vi "fuse_CAN_tester.vi"() -> ()   [LabVIEW 2010]
uses:
  <vilib>/Platform/TimedLoop/XDataNode/XDataNode.xnode
  <vilib>/Platform/TimedLoop/XDataNode/timing_clust.ctl
  <vilib>/Platform/TimedLoop/XDataNode/nitl_modes.ctl
  <vilib>/Platform/TimedLoop/XDataNode/wakeup.ctl
  <vilib>/Platform/TimedLoop/XDataNode/XDNodeRunTimeDep.lvlib
panel:
  in  "Save Params":bool
  in  "Frequancy":i32
  out "WD reset":bool
  in  "Clear buffer":bool
  out "Error number":string
  in  "Get Faults":bool
  out "FF OC":bool
  out "Comperator OC":bool
  out "ADC OC":bool
  in  "Params Menu":u8(ring) items=["Address", "Interval Period", "Nm Of Retries", "On time", "Save Parameters"]
  in  "Send Param":bool
  in  "Repeat Command":bool
  in  "Send":bool
  in  "Command Menu":u8(ring) items=["Status"=0, "ADC Reading"=1, "Isc threshold"=2, "Vin Vout"=15, "RESET FF"=3, "Up Time"=5, "Interval Period"=6, "Nm Of Retries"=7, "On time"=8, "Version"=10, "Temperature"=16]
  out "RT (Ohms)":dbl
  out "Temp (C)":dbl
  out "Vout [V]":dbl
  out "Vin [V]":dbl
  in  "Address":u32
  in  "Interval Period":u32
  in  "Nm. Retries":u32
  in  "On Time [us]":u32
  out "On Time [us]":u32
  out "Nm. Retries":u32
  out "Interval [ms]":u32
  out "Up Time":u32
  out "Fuse Current [A]":dbl
  out "ADC Reading":u32
  out "Isc [A]":dbl
  out "Timeout":bool
  out "R Sense [m]":dbl
  out "Fuse Status":bool
  in  "Clear":bool
  out "Command Buffer":string
  out "status":bool
  out "Message List":string
  in  "Open":bool
  in  "Close":bool
  in  "Quit":bool
  in  "Send Message":bool
  in  "Bit Rate":string="250"
  out "Handle":i32
  in  "Data":u8 format="%x"
  in  "Data 2":u8 format="%x"
  in  "Data 3":u8 format="%x"
  in  "Data 4":u8 format="%x"
  in  "Data 5":u8 format="%x"
  in  "Data 6":u8 format="%x"
  in  "Data 7":u8 format="%x"
  in  "Data 8":u8 format="%x"
  in  "TxID":u32 format="%x"
  in  "Extended":bool
  # "Identifier:"
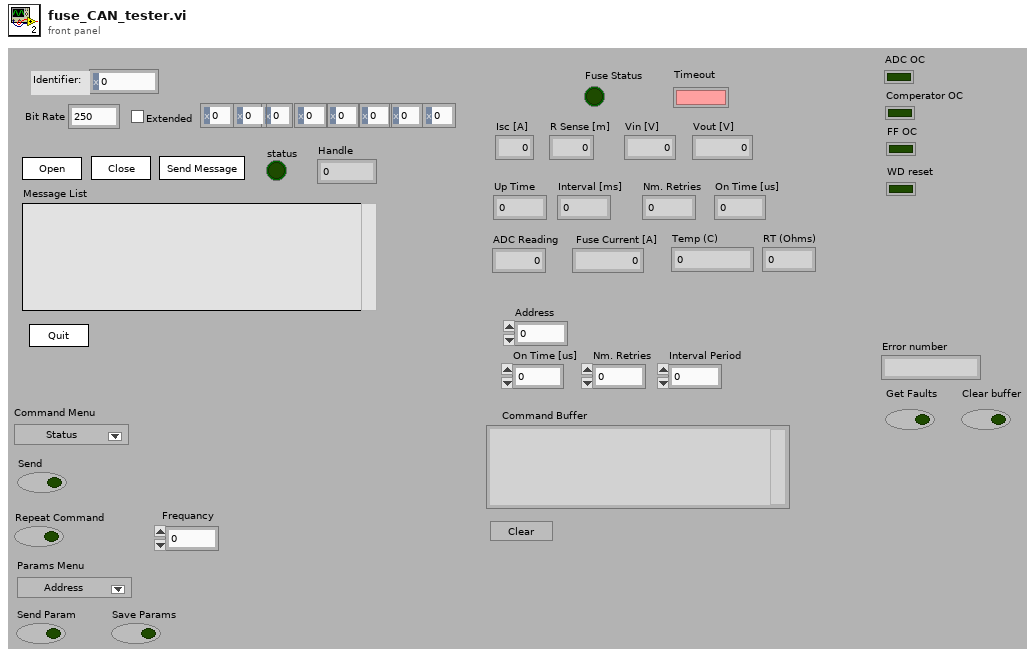
[diagram p1: front panel]
types:
  T1 = typedef "XDNodeRunTimeDep.lvlib/timing_clust.ctl" = cluster{"Expected End [f-1]":u64, "Actual End [f-1]":u64, "Finished Late? [f-1]":bool, "Expected End [i-1]":u64, "Actual End [i-1]":u64, "Finished Late? [i-1]":bool, "Expected Start [i]":u64, "Actual Start [i]":u64, "Expected Start [f]":u64, "Actual Start [f]":u64, "Source Name":string, "Structure Name":string, "Period":i64, "Deadline":i64, "Offset":i64, "Start":i64, "Priority":i32, "Timeout":i32, "Mode":T2, "Wakeup Reason":T3, "Error":errorcluster, "Source Type":string, "Secondary Source Type":string, "Global End Time":u64, "Global Start Time":u64, "Frame Duration":u64, "Iteration Duration":u64, "Assigned CPU":i32, "I/O Scan Engine Mode":u32}
  T2 = typedef "XDNodeRunTimeDep.lvlib/nitl_modes.ctl" = enum32{"No Change", "Process missed periods, maintain original phase", "Discard missed periods, maintain original phase", "Process missed periods, ignore original phase", "Discard missed periods, ignore original phase"}
  T3 = typedef "XDNodeRunTimeDep.lvlib/wakeup.ctl" = enum32{"Normal", "Aborted", "Asynchronous wakeup", "Timing source error", "Timed loop error", "Timeout"}
  T4 = enum32{"invalid app kind", "Development System", "Run Time System", "Student Edition", "Embedded LabVIEW", "Evaluation", "Custom"}
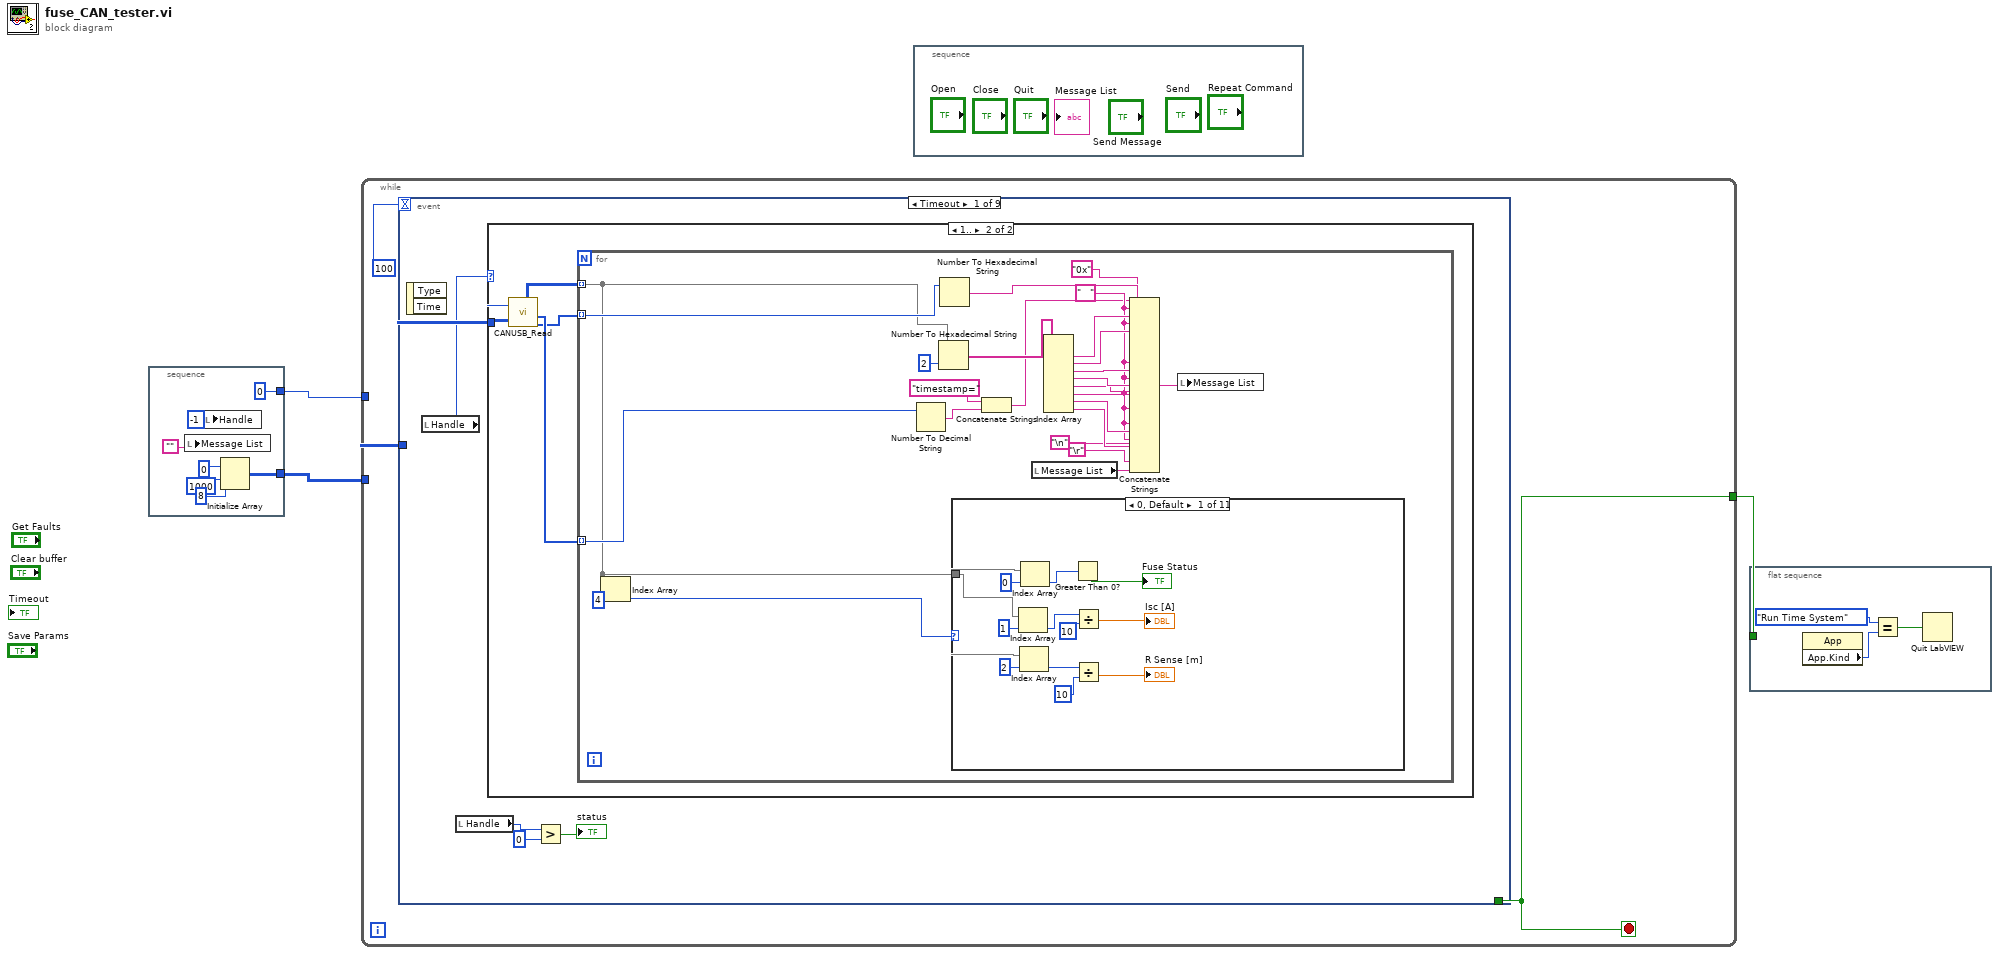
[diagram p0: block diagram]
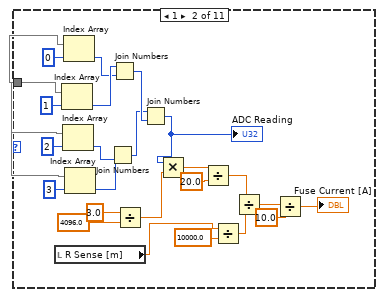
[diagram p3: hidden frame]
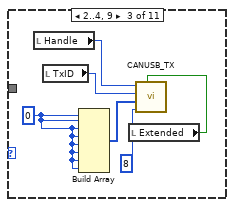
[diagram p4: hidden frame]
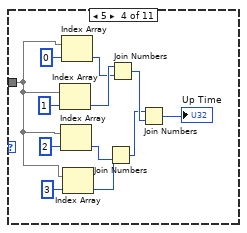
[diagram p5: hidden frame]
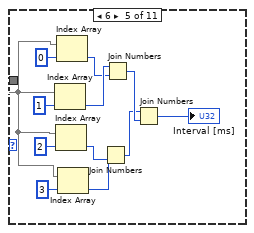
[diagram p6: hidden frame]
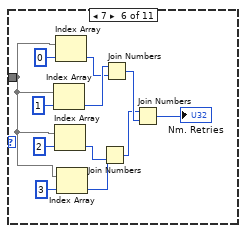
[diagram p7: hidden frame]
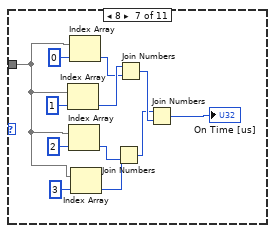
[diagram p8: hidden frame]
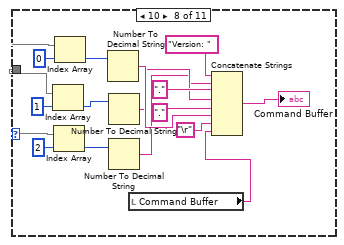
[diagram p9: hidden frame]
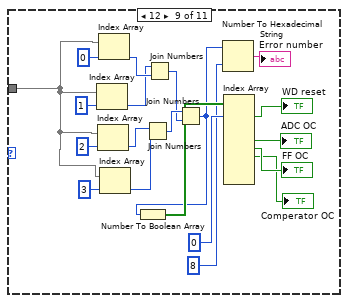
[diagram p10: hidden frame]
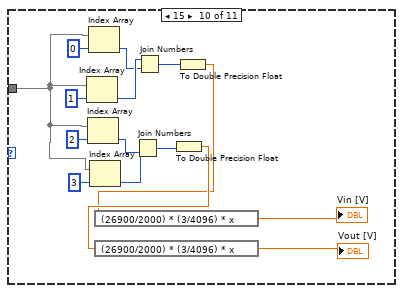
[diagram p11: hidden frame]
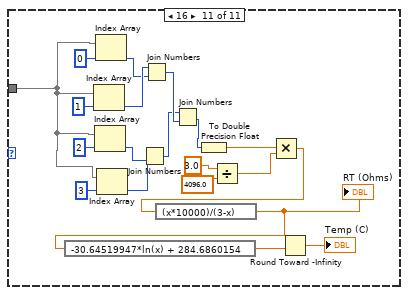
[diagram p12: hidden frame]
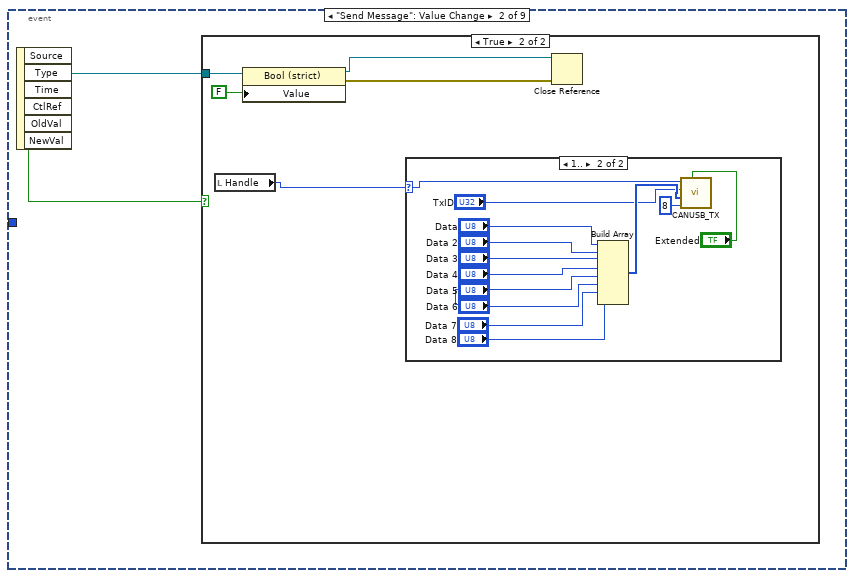
[diagram p13: hidden frame]
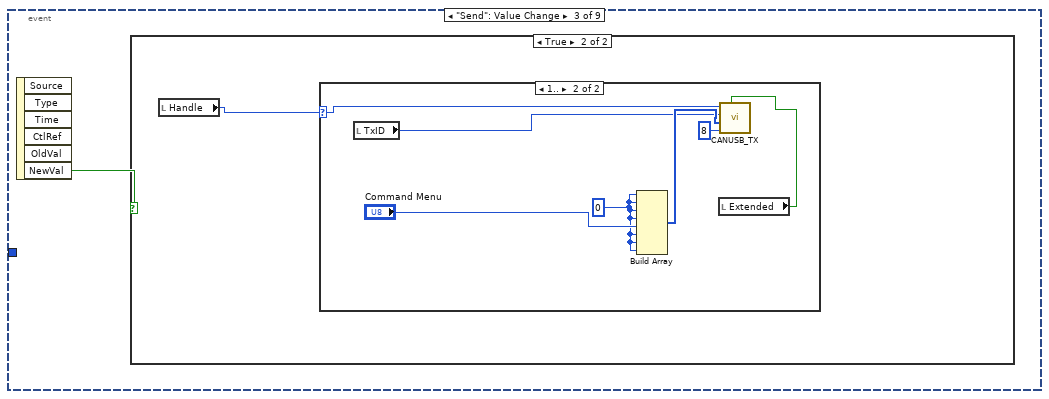
[diagram p16: hidden frame]
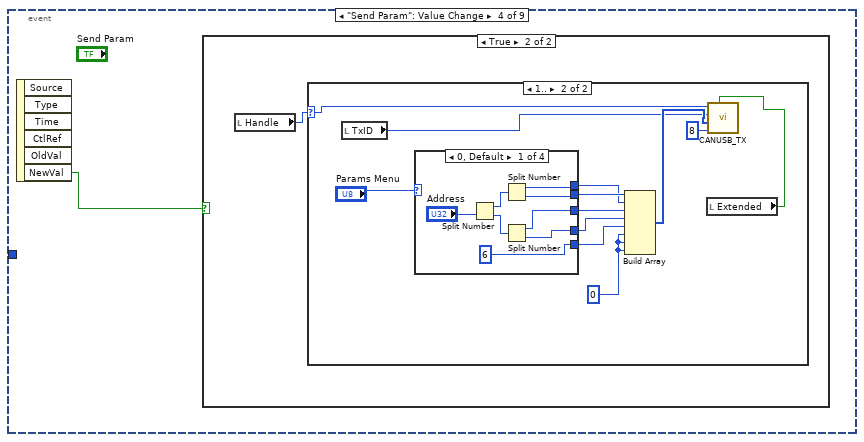
[diagram p19: hidden frame]
diagram:
  n1 = stacked-sequence {
    tunnel: [0] -> w3
    tunnel: [w4] -> w2
    frame #0 {
      n2 = local write "Message List"("") -> ()
      n3 = local write "Handle"(-1 ("Handle")) -> ()
      n4 = Initialize Array(u8 0, 1000 ("dimension size"), 8 ("dimension size")) -> (w4:u8[][])
    }
  }
  n5 = while {
    tunnel: w3 -> [_]
    tunnel: w2 -> [w12]
    tunnel: [w11] -> w1
    stop <- w11 stop-if-true
    n6 = event shown="[0] Timeout" {
      selector: _ -> [_ _ _ _ _ _ _ _ _]
      dyn-events: _ -> [_ _ _ _ _ _ _ _ _]
      timeout: 100 -> [_ _ _ _ _ _ _ _ _]
      tunnel: [_ _ _ _ _ _ _ w330 _] -> w11
      tunnel: w12 -> [w18 _ _ _ _ _ _ _ _]
      event Timeout {
        n7 = event-data() -> ()  [unwired: 1 in, 2 out]
        n8 = local read "Handle"() -> (w17:i32)
        n9 = local read "Handle"() -> (w15:i32)
        n10 = case shown="1.." w17 {
          selector: w17 -> [_ w22]
          tunnel: w18 -> [_ w23]
          frame 0, Default {
          }
          frame 1.. {
            n11 = call "CANUSB_Read.vi"("Buffer"=w23, "handle in"=w22) -> ("ID Array Out"=w19:u32[], "Time Stamps"=w21:u32[], "Data Array Out"=w20:u8[][])  [unwired: 2 out]
            n12 = for {
              tunnel: w21 -> [w28] mode=indexing
              tunnel: w20 -> [w24] mode=indexing
              tunnel: w19 -> [w27] mode=indexing
              w33 = "   " ("string")
              n13 = Index Array(array=w24, index=4) -> (element=w25:u8)
              n14 = Number To Decimal String(number=w28) -> (decimal integer string=w32:string)  [unwired: 1 in]
              n15 = Number To Hexadecimal String(1:i16 2 ("width (-)"), 2:w24) -> (0:w47:string[])
              n16 = Number To Hexadecimal String(2:w27) -> (0:w34:string)  [unwired: 1 in]
              n17 = case shown="0, Default" w25 {
                tunnel: w24 -> [w52 w64 _ w92 w104 w116 w128 w151 w160 w177 w192]
                frame 0, Default {
                  n18 = Index Array(array=w52, index=1) -> (element=w54:u8)
                  n19 = Index Array(array=w52, index=2) -> (element=w56:u8)
                  n20 = Index Array(array=w52, index=0) -> (element=w60:u8)
                  n21 = Greater Than 0?(x=w60) -> (x > 0?=→"Fuse Status":bool)
                  n22 = Divide(x=w54, y=u8 10) -> (x/y=→"Isc [A]":dbl)
                  n23 = Divide(x=w56, y=u8 10) -> (x/y=→"R Sense [m]":dbl)
                }
                frame 1 {
                  n24 = local read "R Sense [m]"() -> (w61:dbl)
                  n25 = Index Array(array=w64, index=1) -> (element=w80:u8)
                  n26 = Index Array(array=w64, index=2) -> (element=w77:u8)
                  n27 = Index Array(array=w64, index=0) -> (element=w79:u8)
                  n28 = Index Array(array=w64, index=3) -> (element=w78:u8)
                  n29 = Join Numbers(hi=w78, lo=w77) -> ((hi.lo)=w75:u16)
                  n30 = Join Numbers(hi=w80, lo=w79) -> ((hi.lo)=w76:u16)
                  n31 = Divide(x=3.0, y=4096.0) -> (x/y=w72:dbl)
                  n32 = Join Numbers(hi=w75, lo=w76) -> ((hi.lo)=w63:u32)
                  "ADC Reading" <- w63
                  n33 = Multiply(x=w63, y=w72) -> (x*y=w71:dbl)
                  n34 = Divide(x=w71, y=20.0) -> (x/y=w69:dbl)
                  n35 = Divide(x=w61, y=10000.0) -> (x/y=w68:dbl)
                  n36 = Divide(x=w69, y=w68) -> (x/y=w66:dbl)
                  n37 = Divide(x=w66, y=10.0) -> (x/y=→"Fuse Current [A]":dbl)
                }
                frame 2..4, 9 {
                  w88 = u8 0 ("element")
                  n38 = local read "Handle"() -> (w85:i32)
                  n39 = local read "TxID"() -> (w90:u32)
                  n40 = Build Array(w88, w88, w88, w88, w88, w88, w88, w88) -> (w87:u8[])
                  n41 = local read "Extended"() -> (w89:bool)
                  n42 = call "CANUSB_TX.vi"("handle in"=w85, "msgID"=w90, "Tx Data"=w87, "Length"=u8 8, "ExtID?"=w89) -> ()  [unwired: 3 out]
                }
                frame 5 {
                  n43 = Index Array(array=w92, index=1) -> (element=w98:u8)
                  n44 = Index Array(array=w92, index=2) -> (element=w95:u8)
                  n45 = Index Array(array=w92, index=0) -> (element=w97:u8)
                  n46 = Index Array(array=w92, index=3) -> (element=w96:u8)
                  n47 = Join Numbers(hi=w96, lo=w95) -> ((hi.lo)=w93:u16)
                  n48 = Join Numbers(hi=w98, lo=w97) -> ((hi.lo)=w94:u16)
                  n49 = Join Numbers(hi=w93, lo=w94) -> ((hi.lo)=→"Up Time":u32)
                }
                frame 6 {
                  n50 = Index Array(array=w104, index=1) -> (element=w110:u8)
                  n51 = Index Array(array=w104, index=2) -> (element=w107:u8)
                  n52 = Index Array(array=w104, index=0) -> (element=w109:u8)
                  n53 = Index Array(array=w104, index=3) -> (element=w108:u8)
                  n54 = Join Numbers(hi=w108, lo=w107) -> ((hi.lo)=w105:u16)
                  n55 = Join Numbers(hi=w110, lo=w109) -> ((hi.lo)=w106:u16)
                  n56 = Join Numbers(hi=w105, lo=w106) -> ((hi.lo)=→"Interval [ms]":u32)
                }
                frame 7 {
                  n57 = Index Array(array=w116, index=1) -> (element=w122:u8)
                  n58 = Index Array(array=w116, index=2) -> (element=w119:u8)
                  n59 = Index Array(array=w116, index=0) -> (element=w121:u8)
                  n60 = Index Array(array=w116, index=3) -> (element=w120:u8)
                  n61 = Join Numbers(hi=w120, lo=w119) -> ((hi.lo)=w117:u16)
                  n62 = Join Numbers(hi=w122, lo=w121) -> ((hi.lo)=w118:u16)
                  n63 = Join Numbers(hi=w117, lo=w118) -> ((hi.lo)=→"Nm. Retries":u32)
                }
                frame 8 {
                  n64 = Index Array(array=w128, index=1) -> (element=w134:u8)
                  n65 = Index Array(array=w128, index=2) -> (element=w131:u8)
                  n66 = Index Array(array=w128, index=0) -> (element=w133:u8)
                  n67 = Index Array(array=w128, index=3) -> (element=w132:u8)
                  n68 = Join Numbers(hi=w132, lo=w131) -> ((hi.lo)=w129:u16)
                  n69 = Join Numbers(hi=w134, lo=w133) -> ((hi.lo)=w130:u16)
                  n70 = Join Numbers(hi=w129, lo=w130) -> ((hi.lo)=→"On Time [us]":u32)
                }
                frame 10 {
                  n71 = Index Array(array=w151, index=1) -> (element=w149:u8)
                  n72 = Index Array(array=w151, index=2) -> (element=w148:u8)
                  n73 = Index Array(array=w151, index=0) -> (element=w150:u8)
                  n74 = Number To Decimal String(number=w150) -> (decimal integer string=w143:string)  [unwired: 1 in]
                  n75 = Number To Decimal String(number=w149) -> (decimal integer string=w142:string)  [unwired: 1 in]
                  n76 = Number To Decimal String(number=w148) -> (decimal integer string=w141:string)  [unwired: 1 in]
                  n77 = local read "Command Buffer"() -> (w139:string)
                  n78 = Concatenate Strings("Version: " ("string"), w141, "." ("string"), w142, "." ("string"), w143, "\r", w139) -> (→"Command Buffer":string)
                }
                frame 12 {
                  n79 = Index Array(array=w160, index=1) -> (element=w165:u8)
                  n80 = Index Array(array=w160, index=2) -> (element=w168:u8)
                  n81 = Index Array(array=w160, index=0) -> (element=w166:u8)
                  n82 = Index Array(array=w160, index=3) -> (element=w167:u8)
                  n83 = Join Numbers(hi=w167, lo=w168) -> ((hi.lo)=w170:u16)
                  n84 = Join Numbers(hi=w165, lo=w166) -> ((hi.lo)=w169:u16)
                  n85 = Join Numbers(hi=w170, lo=w169) -> ((hi.lo)=w172:u32)
                  n86 = Number To Boolean Array(number=w172) -> (Boolean array=w173:bool[])
                  n87 = Number To Hexadecimal String(1:i16 8 ("width (-)"), 2:w172) -> (0:→"Error number":string)
                  n88 = Index Array(array=w173, index #1=0 ("index")) -> (element #1=→"WD reset":bool, element #4=→"ADC OC":bool, element #5=→"FF OC":bool, element #6=→"Comperator OC":bool)  [unwired: 8 in, 5 out]
                }
                frame 15 {
                  n89 = Index Array(array=w177, index=1) -> (element=w185:u8)
                  n90 = Index Array(array=w177, index=2) -> (element=w182:u8)
                  n91 = Index Array(array=w177, index=0) -> (element=w184:u8)
                  n92 = Index Array(array=w177, index=3) -> (element=w183:u8)
                  n93 = Join Numbers(hi=w183, lo=w182) -> ((hi.lo)=w180:u16)
                  n94 = Join Numbers(hi=w185, lo=w184) -> ((hi.lo)=w181:u16)
                  n95 = To Double Precision Float(number=w180) -> (double precision float=w179:dbl)
                  n96 = expression code="(26900/2000) * (3/4096) * x"(w179) -> (→"Vout [V]":dbl)
                  n97 = To Double Precision Float(number=w181) -> (double precision float=w178:dbl)
                  n98 = expression code="(26900/2000) * (3/4096) * x"(w178) -> (→"Vin [V]":dbl)
                }
                frame 16 {
                  n99 = Index Array(array=w192, index=1) -> (element=w205:u8)
                  n100 = Index Array(array=w192, index=2) -> (element=w202:u8)
                  n101 = Index Array(array=w192, index=0) -> (element=w204:u8)
                  n102 = Index Array(array=w192, index=3) -> (element=w203:u8)
                  n103 = Join Numbers(hi=w203, lo=w202) -> ((hi.lo)=w200:u16)
                  n104 = Join Numbers(hi=w205, lo=w204) -> ((hi.lo)=w201:u16)
                  n105 = Join Numbers(hi=w200, lo=w201) -> ((hi.lo)=w199:u32)
                  n106 = To Double Precision Float(number=w199) -> (double precision float=w195:dbl)
                  n107 = Divide(x=3.0, y=4096.0) -> (x/y=w198:dbl)
                  n108 = Multiply(x=w195, y=w198) -> (x*y=w194:dbl)
                  n109 = expression code="(x*10000)/(3-x)"(w194) -> (w190:dbl)
                  "RT (Ohms)" <- w190
                  n110 = expression code="-30.64519947*ln(x) + 284.6860154"(w190) -> (w193:dbl)
                  n111 = Round Toward -Infinity(1:w193) -> (0:→"Temp (C)":dbl)
                }
              }
              n112 = Concatenate Strings("timestamp=" ("string"), w32) -> (w31:string)
              n113 = local read "Message List"() -> (w38:string)
              n114 = Index Array(array=w47) -> (element #1=w46:string, element #2=w45:string, element #3=w44:string, element #4=w43:string, element #5=w42:string, element #6=w41:string, element #7=w40:string, element #8=w39:string)  [unwired: 8 in]
              n115 = Concatenate Strings("0x", w34, w33, w31, w33, w46, w33, w45, w33, w44, w33, w43, w33, w42, w33, w41, w33, w40, w33, w39, "\n", "\r", w38) -> (w48:string)
              n116 = local write "Message List"(w48) -> ()
            }
          }
        }
        n117 = Greater?(x=w15, y=0) -> (0:→"status":bool)
      }
      event "Send Message": Value Change {
        n118 = event-data() -> ("CtlRef"=w210:refnum<vi>, "NewVal"=w211:bool)  [unwired: 1 in, 4 out]
        n119 = case shown="True" w211 {
          tunnel: w210 -> [_ w216]
          frame False {
          }
          frame True {
            n120 = local read "Handle"() -> (w212:i32)
            n121 = property class="Bool (strict)"(reference=w216, "Value"=FALSE) -> (reference out=w213:refnum<vi>, error out=w214:errorcluster)  [unwired: 1 in]
            n122 = case shown="1.." w212 {
              selector: w212 -> [_ w229]
              frame 0, Default {
              }
              frame 1.. {
                n123 = Build Array("Data", "Data 2", "Data 3", "Data 4", "Data 5", "Data 6", "Data 7", "Data 8") -> (w220:u8[])
                n124 = call "CANUSB_TX.vi"("handle in"=w229, "msgID"="TxID", "Tx Data"=w220, "Length"=u8 8, "ExtID?"="Extended") -> ()  [unwired: 3 out]
              }
            }
            n125 = Close Reference(reference=w213, error in (no error)=w214) -> ()  [unwired: 1 out]
          }
        }
      }
      event "Send": Value Change {
        n126 = event-data() -> ("NewVal"=w230:bool)  [unwired: 1 in, 5 out]
        n127 = case shown="True" w230 {
          frame False {
          }
          frame True {
            n128 = local read "Handle"() -> (w231:i32)
            n129 = case shown="1.." w231 {
              selector: w231 -> [_ w238]
              frame 0, Default {
              }
              frame 1.. {
                w233 = u8 0 ("element")
                n130 = local read "TxID"() -> (w235:u32)
                n131 = Build Array(w233, w233, w233, w233, "Command Menu", w233, w233, w233) -> (w237:u8[])
                n132 = local read "Extended"() -> (w232:bool)
                n133 = call "CANUSB_TX.vi"("handle in"=w238, "msgID"=w235, "Tx Data"=w237, "Length"=u8 8, "ExtID?"=w232) -> ()  [unwired: 3 out]
              }
            }
          }
        }
      }
      event "Send Param": Value Change {
        n134 = event-data() -> ("NewVal"=w239:bool)  [unwired: 1 in, 5 out]
        n135 = case shown="True" w239 {
          frame False {
          }
          frame True {
            n136 = local read "Handle"() -> (w240:i32)
            n137 = case shown="1.." w240 {
              selector: w240 -> [_ w252]
              frame 0, Default {
              }
              frame 1.. {
                w246 = u8 0 ("element")
                n138 = local read "TxID"() -> (w249:u32)
                n139 = case shown="0, Default" "Params Menu" {
                  tunnel: [u8 6 ("element") u8 6 ("element") u8 7 ("element") u8 8 ("element")] -> w245
                  tunnel: [w256 w264 w273 w281] -> w244
                  tunnel: [w257 w263 w274 w282] -> w243
                  tunnel: [w255 w262 w272 w280] -> w242
                  tunnel: [w254 w261 w271 w279] -> w241
                  frame 0, Default {
                    n140 = Split Number(x="Address") -> (hi(x)=w258:u16, lo(x)=w260:u16)
                    n141 = Split Number(x=w258) -> (hi(x)=w257:u8, lo(x)=w256:u8)
                    n142 = Split Number(x=w260) -> (hi(x)=w255:u8, lo(x)=w254:u8)
                  }
                  frame 1 {
                    n143 = Split Number(x="Interval Period") -> (hi(x)=w268:u16, lo(x)=w267:u16)
                    n144 = Split Number(x=w268) -> (hi(x)=w264:u8, lo(x)=w263:u8)
                    n145 = Split Number(x=w267) -> (hi(x)=w262:u8, lo(x)=w261:u8)
                  }
                  frame 2 {
                    n146 = Split Number(x="Nm. Retries") -> (hi(x)=w275:u16, lo(x)=w276:u16)
                    n147 = Split Number(x=w275) -> (hi(x)=w274:u8, lo(x)=w273:u8)
                    n148 = Split Number(x=w276) -> (hi(x)=w272:u8, lo(x)=w271:u8)
                  }
                  frame 3 {
                    n149 = Split Number(x="On Time [us]") -> (hi(x)=w283:u16, lo(x)=w284:u16)
                    n150 = Split Number(x=w283) -> (hi(x)=w282:u8, lo(x)=w281:u8)
                    n151 = Split Number(x=w284) -> (hi(x)=w280:u8, lo(x)=w279:u8)
                  }
                }
                n152 = Build Array(w244, w243, w242, w241, w245, w246, w246, w246) -> (w251:u8[])
                n153 = local read "Extended"() -> (w248:bool)
                n154 = call "CANUSB_TX.vi"("handle in"=w252, "msgID"=w249, "Tx Data"=w251, "Length"=u8 8, "ExtID?"=w248) -> ()  [unwired: 3 out]
              }
            }
          }
        }
      }
      event "Repeat Command": Value Change {
        n155 = event-data() -> ("NewVal"=w286:bool)  [unwired: 1 in, 5 out]
        n156 = Not(x=w286) -> (.not. x?=w285:bool)
        n157 = node-c288("Frequancy") -> (w289:T1)  [unwired: 3 in]
        n158 = timed-loop {
          timing: w289 -> [_]
          timing-out: [_] -> w288
          tunnel: w285 -> [w290]
          stop <- w290 stop-if-true
          n159 = node-c288() -> ()  [unwired: 1 in, 1 out]
          n160 = local read "Handle"() -> (w291:i32)
          n161 = case shown="1.." w291 {
            selector: w291 -> [_ w298]
            frame 0, Default {
            }
            frame 1.. {
              w294 = u8 0 ("element")
              n162 = local read "Command Menu"() -> (w292:u8)
              n163 = local read "TxID"() -> (w295:u32)
              n164 = Build Array(w294, w294, w294, w294, w292, w294, w294, w294) -> (w297:u8[])
              n165 = local read "Extended"() -> (w293:bool)
              n166 = call "CANUSB_TX.vi"("handle in"=w298, "msgID"=w295, "Tx Data"=w297, "Length"=u8 8, "ExtID?"=w293) -> ()  [unwired: 3 out]
            }
          }
          n167 = node-c288() -> ()  [unwired: 1 in, 1 out]
        }
        n168 = node-c288(w288) -> ()  [unwired: 1 out]
      }
      event "Open": Value Change {
        n169 = event-data() -> ("CtlRef"=w305:refnum<vi>, "NewVal"=w306:bool)  [unwired: 1 in, 4 out]
        n170 = case shown="True" w306 {
          tunnel: w305 -> [_ w311]
          frame False {
          }
          frame True {
            n171 = local read "Handle"() -> (w307:i32)
            n172 = property class="Bool (strict)"(reference=w311, "Value"=FALSE) -> (reference out=w309:refnum<vi>, error out=w308:errorcluster)  [unwired: 1 in]
            n173 = case shown="0, Default" w307 {
              frame 0, Default {
                n174 = call "CANUSB_Open.vi"("acceptance_mask"=u32 4294967295, "acceptance_code"=u32 0, "szBitrate"="Bit Rate") -> ("verinfo"=w313:string, "Handle"=→"Handle":i32)  [unwired: 3 in, 1 out]
                n175 = local read "Message List"() -> (w312:string)
                n176 = Concatenate Strings(w313, "\n", "\r", w312) -> (w316:string)
                n177 = local write "Message List"(w316) -> ()
              }
              frame 1.. {
              }
            }
            n178 = Close Reference(reference=w309, error in (no error)=w308) -> ()  [unwired: 1 out]
          }
        }
      }
      event "Close": Value Change {
        n179 = event-data() -> ("CtlRef"=w321:refnum<vi>, "NewVal"=w322:bool)  [unwired: 1 in, 4 out]
        n180 = case shown="True" w322 {
          tunnel: w321 -> [_ w327]
          frame False {
          }
          frame True {
            n181 = local read "Handle"() -> (w323:i32)
            n182 = property class="Bool (strict)"(reference=w327, "Value"=FALSE) -> (reference out=w325:refnum<vi>, error out=w324:errorcluster)  [unwired: 1 in]
            n183 = case shown="1.." w323 {
              selector: w323 -> [_ w329]
              frame 0, Default {
              }
              frame 1.. {
                n184 = call "CANUSB_Close.vi"("Handle"=w329) -> ()  [unwired: 1 out]
                n185 = local write "Handle"(-1 ("Handle")) -> ()
              }
            }
            n186 = Close Reference(reference=w325, error in (no error)=w324) -> ()  [unwired: 1 out]
          }
        }
      }
      event "Quit": Value Change {
        n187 = event-data() -> ("CtlRef"=w331:refnum<vi>, "NewVal"=w332:bool)  [unwired: 1 in, 4 out]
        n188 = case shown="True" w332 {
          tunnel: w331 -> [_ w339]
          tunnel: [FALSE w334] -> w330
          frame False {
          }
          frame True {
            n189 = local read "Handle"() -> (w335:i32)
            n190 = property class="Bool (strict)"(reference=w339, "Value"=FALSE) -> (reference out=w337:refnum<vi>, error out=w336:errorcluster)  [unwired: 1 in]
            n191 = case shown="0, Default" w335 {
              selector: w335 -> [_ w342]
              tunnel: [TRUE TRUE] -> w334
              frame 0, Default {
              }
              frame 1.. {
                n192 = call "CANUSB_Close.vi"("Handle"=w342) -> ()  [unwired: 1 out]
              }
            }
            n193 = Close Reference(reference=w337, error in (no error)=w336) -> ()  [unwired: 1 out]
          }
        }
      }
      event "Clear": Value Change {
        n194 = event-data() -> ()  [unwired: 1 in, 5 out]
        n195 = local write "Command Buffer"("" ("Command Buffer")) -> ()
      }
    }
  }
  n196 = stacked-sequence {
    frame #0 {
    }
  }
  n197 = flat-sequence {
    tunnel: w1 -> [_]
    frame #0 {
      n198 = property class="App"() -> ("App.Kind"=w345:T4)  [unwired: 2 in, 2 out]
      n199 = Equal?(x=T4."Run Time System" ("Application:Kind"), y=w345) -> (x = y?=w344:bool)
      n200 = Quit LabVIEW(quit? (T)=w344) -> ()
    }
  }
